vi "Color-Senser-Correction_Api.vi"(5 "加速度":i32=400, 6 "觸發數值":dbl=90.0 format="%#_13g", 7 "最高速":i32=400, 8 "Error In":errorcluster, 11 "接收位置":dbl format="%#_13g") -> (0 "Error Out":errorcluster)   [LabVIEW 2019]
uses:
  <vilib>/Platform/TimedLoop/XDataNode/timing_clust.ctl
  <vilib>/Platform/TimedLoop/XDataNode/nitl_modes.ctl
  <vilib>/Platform/TimedLoop/XDataNode/wakeup.ctl
  <vilib>/platform/TimedLoop/XDataNode/XDataNode.xnode
  <vilib>/Platform/TimedLoop/XDataNode/XDNodeRunTimeDep.lvlib
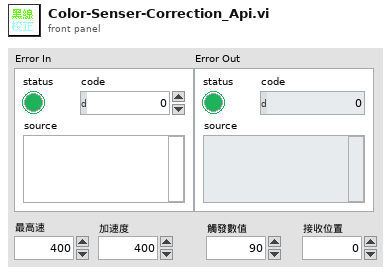
[diagram p1: front panel]
types:
  T1 = typedef "XDNodeRunTimeDep.lvlib/timing_clust.ctl" = cluster{"Expected End [f-1]":u64, "Actual End [f-1]":u64, "Finished Late? [f-1]":bool, "Expected End [i-1]":u64, "Actual End [i-1]":u64, "Finished Late? [i-1]":bool, "Expected Start [i]":u64, "Actual Start [i]":u64, "Expected Start [f]":u64, "Actual Start [f]":u64, "Source Name":string, "Structure Name":string, "Period":i64, "Deadline":i64, "Offset":i64, "Start":i64, "Priority":i32, "Timeout":i32, "Mode":T2, "Wakeup Reason":T3, "Error":errorcluster, "Source Type":string, "Secondary Source Type":string, "Global End Time":u64, "Global Start Time":u64, "Frame Duration":u64, "Iteration Duration":u64, "Assigned CPU":i32, "I/O Scan Engine Mode":u32}
  T2 = typedef "XDNodeRunTimeDep.lvlib/nitl_modes.ctl" = enum32{"No Change", "Process missed periods, maintain original phase", "Discard missed periods, maintain original phase", "Process missed periods, ignore original phase", "Discard missed periods, ignore original phase"}
  T3 = typedef "XDNodeRunTimeDep.lvlib/wakeup.ctl" = enum32{"Normal", "Aborted", "Asynchronous wakeup", "Timing source error", "Timed loop error", "Timeout"}
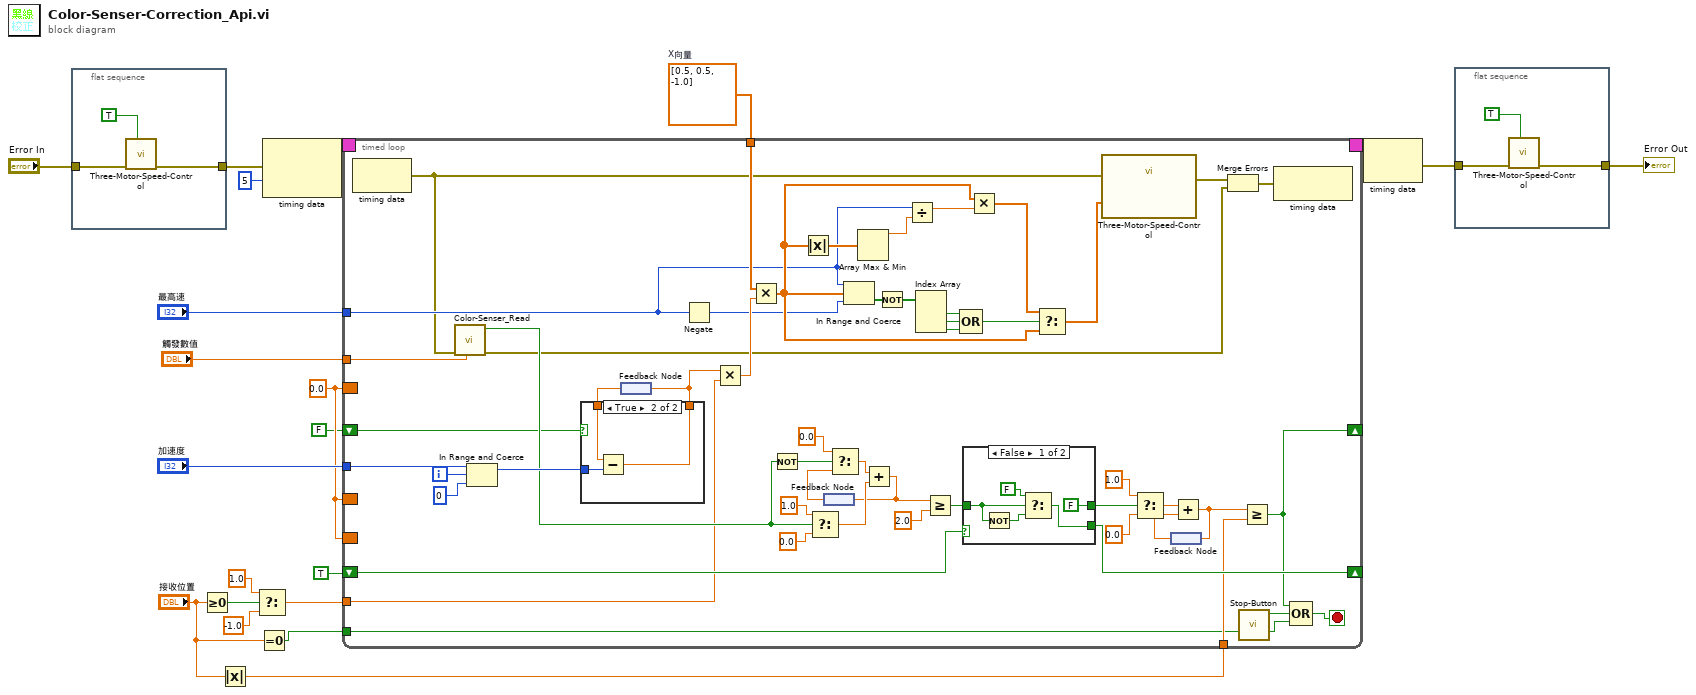
[diagram p0: block diagram]
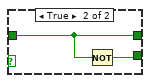
[diagram p2: hidden frame]
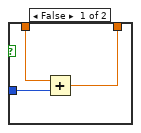
[diagram p3: hidden frame]
diagram:
  w13 = 0.0
  w18 = dbl[] [0.5, 0.5, -1.0]  # X向量
  n1 = flat-sequence {
    tunnel: [w24] -> w6
    tunnel: "Error In" -> [w22]
    frame #0 {
      n2 = call "Three-Motor-Speed-Control.vi"("Reset"=TRUE, "Error In"=w22) -> ("Error Out"=w24:errorcluster)  [unwired: 9 in]
    }
  }
  n3 = Greater Or Equal To 0?(x="接收位置") -> (x >= 0?=w12:bool)
  n4 = Absolute Value(x="接收位置") -> (abs(x)=w8:dbl)
  n5 = Select(t=1.0, s=w12, f=-1.0) -> (s? t:f=w9:dbl)
  n6 = Equal To 0?(x="接收位置") -> (x = 0?=w4:bool)
  n7 = node-c288(w6, i64 5 ("Period")) -> (w21:T1)
  n8 = timed-loop {
    timing: w21 -> [_]
    timing-out: [_] -> w20
    tunnel: w18 -> [w76]
    tunnel: "觸發數值" -> [w51]
    tunnel: "加速度" -> [w73]
    tunnel: "最高速" -> [w31]
    border: w13 -> [_]
    border: w13 -> [_]
    border: w13 -> [_]
    shift-right: [w55] -> _
    shift-left: TRUE -> [w58]
    tunnel: w9 -> [w47]
    tunnel: w8 -> [w50]
    tunnel: w4 -> [w46]
    shift-right: [w26] -> _
    shift-left: FALSE -> [w25]
    i -> [w75]
    stop <- w77 stop-if-true
    n9 = node-c288() -> (w30:errorcluster)  [unwired: 1 in]
    n10 = call "Color-Senser_Read.vi"("觸發數值"=w51, "Error In"=w30) -> ("Error Out"=w27:errorcluster, "觸發?"=w49:bool)  [unwired: 7 in, 1 out]
    n11 = In Range and Coerce(upper limit=w73, x=w75, lower limit=0) -> (coerced(x)=w54:i32)  [unwired: 1 out]
    n12 = feedback #1() -> (w72:dbl)
    n13 = case shown="True" w25 {
      tunnel: w54 -> [w92 w95]
      tunnel: [w91 w93] -> w48
      tunnel: w72 -> [w90 w94]
      frame False {
        n14 = Add(x=w90, y=w92) -> (x+y=w91:dbl)
      }
      frame True {
        n15 = Subtract(x=w94, y=w95) -> (x-y=w93:dbl)
      }
    }
    n16 = feedback-in #1(w48) -> ()
    n17 = Negate(x=w31) -> (-x=w32:i32)
    n18 = Multiply(x=w48, y=w47) -> (x*y=w45:dbl)
    n19 = Multiply(x=w76, y=w45) -> (x*y=w34:dbl[])
    n20 = Not(x=w49) -> (.not. x?=w68:bool)
    n21 = Absolute Value(x=w34) -> (abs(x)=w35:dbl[])
    n22 = Select(t=1.0, s=w49, f=0.0) -> (s? t:f=w70:dbl)
    n23 = feedback #2() -> (w69:dbl)
    n24 = Select(t=0.0, s=w68, f=w69) -> (s? t:f=w66:dbl)
    n25 = In Range and Coerce(upper limit=w31, x=w34, lower limit=w32) -> (In Range?=w44:bool[])  [unwired: 1 out]
    n26 = Array Max & Min(array=w35) -> (max value=w36:dbl)  [unwired: 3 out]
    n27 = Add(x=w66, y=w70) -> (x+y=w65:dbl)
    n28 = feedback-in #2(w65) -> ()
    n29 = Not(x=w44) -> (.not. x?=w43:bool[])
    n30 = Divide(x=w31, y=w36) -> (x/y=w38:dbl)
    n31 = Index Array(array=w43) -> (element #1=w42:bool, element #2=w41:bool, element #3=w40:bool)  [unwired: 3 in]
    n32 = Greater Or Equal?(x=w65, y=2.0) -> (x >= y?=w57:bool)
    n33 = Compound Arithmetic op=OR(w42, w41, w40) -> (w39:bool)
    n34 = case shown="False" w58 {
      tunnel: w57 -> [w83 w88]
      tunnel: [FALSE w88] -> w56
      tunnel: [w86 w89] -> w55
      frame False {
        n35 = Not(x=w83) -> (.not. x?=w84:bool)
        n36 = Select(t=FALSE, s=w83, f=w84) -> (s? t:f=w86:bool)
      }
      frame True {
        n37 = Not(x=w88) -> (.not. x?=w89:bool)
      }
    }
    n38 = Multiply(x=w34, y=w38) -> (x*y=w37:dbl[])
    n39 = Select(t=w37, s=w39, f=w34) -> (s? t:f=w33:dbl[])
    n40 = call "Three-Motor-Speed-Control.vi"("Error In"=w30, "速度(秒/度)"=w33) -> ("Error Out"=w28:errorcluster)  [unwired: 9 in]
    n41 = Select(t=1.0, s=w56, f=0.0) -> (s? t:f=w59:dbl)
    n42 = feedback #3() -> (w60:dbl)
    n43 = Add(x=w59, y=w60) -> (x+y=w53:dbl)
    n44 = feedback-in #3(w53) -> ()
    n45 = Merge Errors(w28, w27) -> (w29:errorcluster)
    n46 = call "Stop-Button.vi"() -> ("顯示按下?"=w52:bool)  [unwired: 10 in, 1 out]
    n47 = Greater Or Equal?(x=w53, y=w50) -> (x >= y?=w26:bool)
    n48 = node-c288(w29) -> ()  [unwired: 1 out]
    n49 = Compound Arithmetic op=OR(w26, w52, w46) -> (w77:bool)
  }
  n50 = node-c288(w20) -> (w7:errorcluster)
  n51 = flat-sequence {
    tunnel: w7 -> [w98]
    tunnel: [w97] -> w3
    frame #0 {
      n52 = call "Three-Motor-Speed-Control.vi"("Reset"=TRUE, "Error In"=w98) -> ("Error Out"=w97:errorcluster)  [unwired: 9 in]
    }
  }
  "Error Out" <- w3
